vi "Modbus PLC Comm Tester_Watch Entry Popup.vi"(10 "Reference Format":u16(ring)=6 items=["4 Digits"=4, "5 Digits"=5, "6 Digits"=6], 11 "Entry in":T1) -> (3 "Entry out":T1)   [LabVIEW 2018]
uses:
  Types/Reference Types_Enum.ctl
  MB PLC Client.lvlib
  4fdbb896-3cd3-4ae7-af4f-e8b1f6b38b66.vi
panel:
  in  "Cancel":bool
  in  "OK":bool
  out "Register Type":string
  in  "Name":string
  in  "Data Type":T2(ring)
  in  "Starting Reference":u32
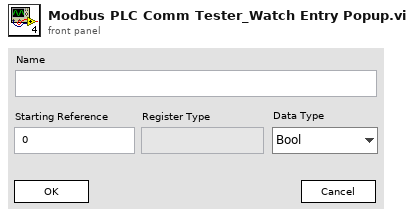
[diagram p1: front panel]
types:
  T1 = cluster{"Name":string, "Reference":u32, "Data Type":enum16{"Bool", "U16", "U32", "I16", "I32", "SGL", "DBL"}}
  T2 = enum16{"Bool", "U16", "U32", "I16", "I32", "SGL", "DBL"}
  T3 = typedef "MB PLC Client.lvlib/Reference Types_Enum.ctl" = enum16{"Coil", "Discrete Input", "Input Register", "Holding Register", "Invalid"}
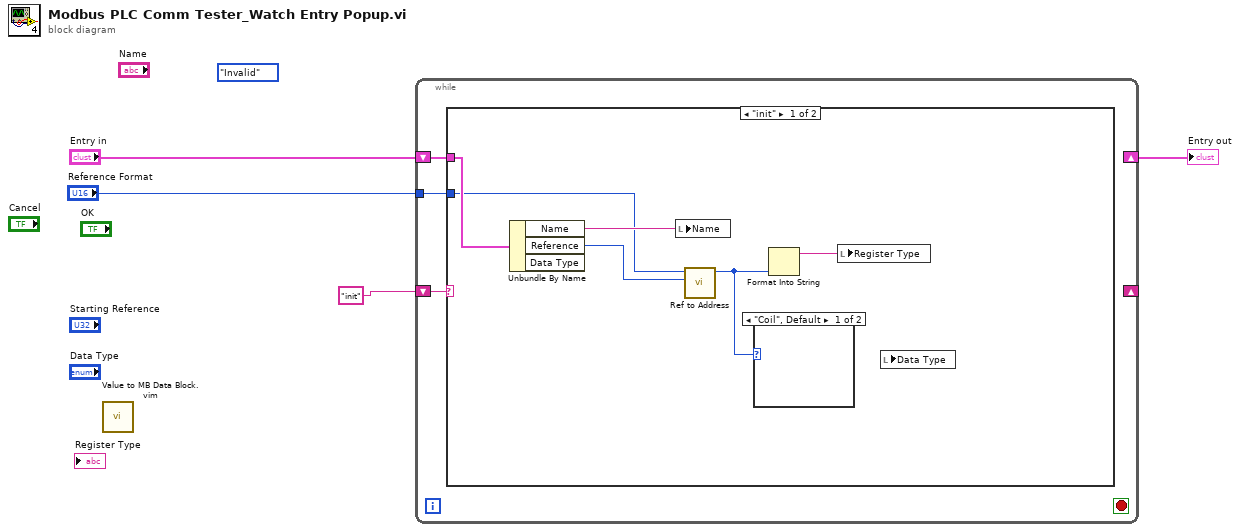
[diagram p0: block diagram]
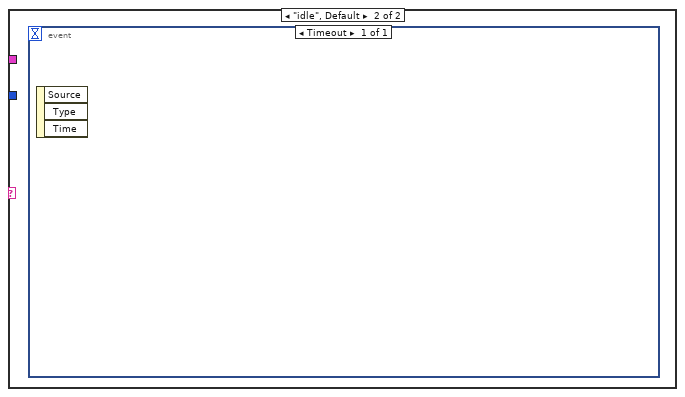
[diagram p3: hidden frame]
diagram:
  w5 = Reference_Types_Enum."Invalid" ("Reference Type")
  n1 = call "Value to MB Data Block.vim"() -> ()  [unwired: 11 in, 1 out]
  n2 = while {
    shift-right: _ -> [_]
    shift-left: "init" -> [w8]
    shift-right: [_] -> w2
    shift-left: "Entry in" -> [w7]
    tunnel: "Reference Format" -> [w6]
    stop <- _ stop-if-true
    n3 = case shown="\"init\"" w8 {
      tunnel: w7 -> [w14 _]
      tunnel: w6 -> [w12 _]
      frame "init" {
        n4 = Unbundle By Name(w14) -> ("Name"=w13:string, "Reference"=w11:u32)  [unwired: 1 out]
        n5 = local write "Name"(w13) -> ()
        n6 = call "Ref to Address.vi"("Reference"=w11, "Reference Format"=w12) -> ("Reference Type"=w9:T3)  [unwired: 8 in, 1 out]
        n7 = case shown="\"Coil\", Default" w9 {
          frame "Coil", Default {
          }
          frame "Discrete Input" {
          }
        }
        n8 = Format Into String(w9) -> (resulting string=w10:string)  [unwired: 3 in, 1 out]
        n9 = local write "Register Type"(w10) -> ()
        n10 = local read "Data Type"() -> ()  [unwired: 1 in]
      }
      frame "idle", Default {
        n11 = event shown="[0] Timeout" {
          selector: _ -> [_]
          dyn-events: _ -> [_]
          timeout: _ -> [_]
          event Timeout {
            n12 = event-data() -> ()  [unwired: 1 in, 3 out]
          }
        }
      }
    }
  }
  "Entry out" <- w2
